vi "DataBase_Main.vi"(8 "error in (no error)":errorcluster) -> (0 "error out":errorcluster)   [LabVIEW 2020]
uses:
  Controller/#typedef_ControllerQueue_States.ctl
panel:
  out "appended path":path
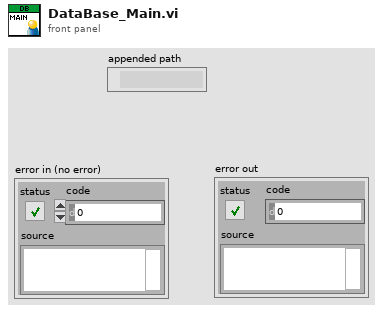
[diagram p1: front panel]
types:
  T1 = typedef "#typedef_ControllerQueue_States.ctl" = enum16{"Obtain", "GetRef", "Enqueue", "EnqueueAtOpp", "GetStatus", "Flush", "Release"}
  T2 = enum16{"open", "replace", "create", "open or create", "replace or create", "replace or create with confirmation"}
  T3 = typedef "#typedef_DataBase.ctl" = cluster{"Cmd":enum16{"Idle", "WriteLog", "Exit"}, "Temperature":dbl, "Logs":string}
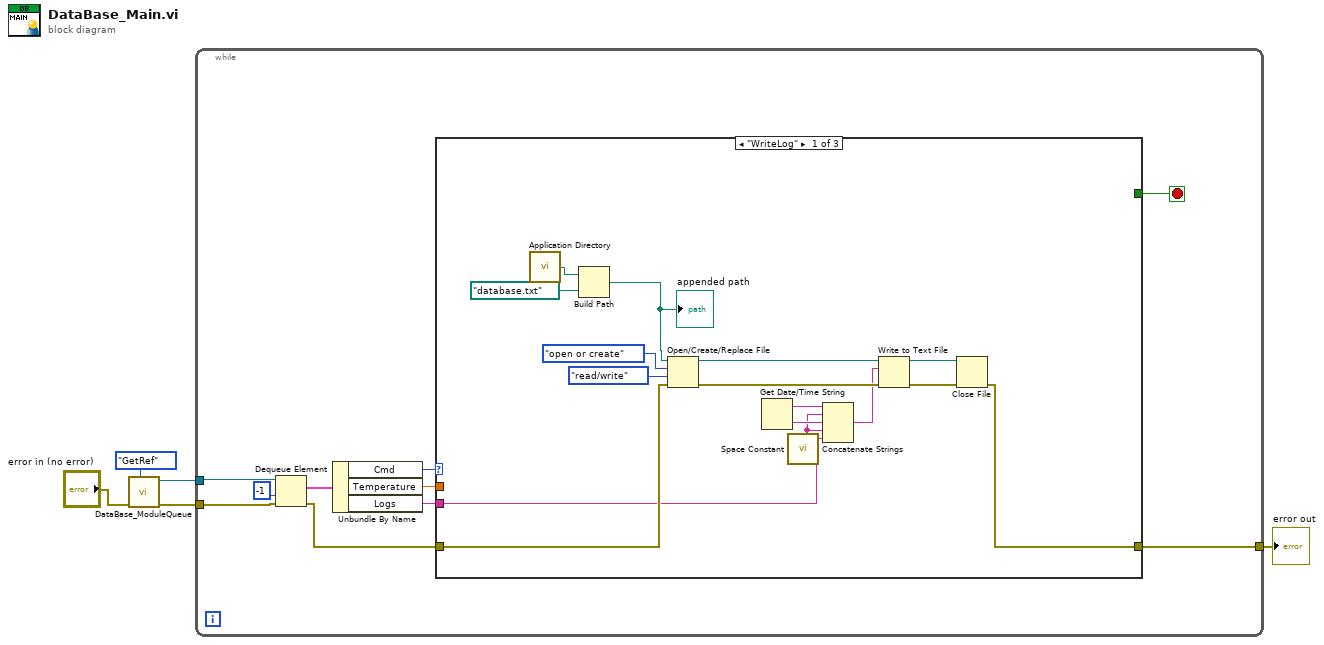
[diagram p0: block diagram]
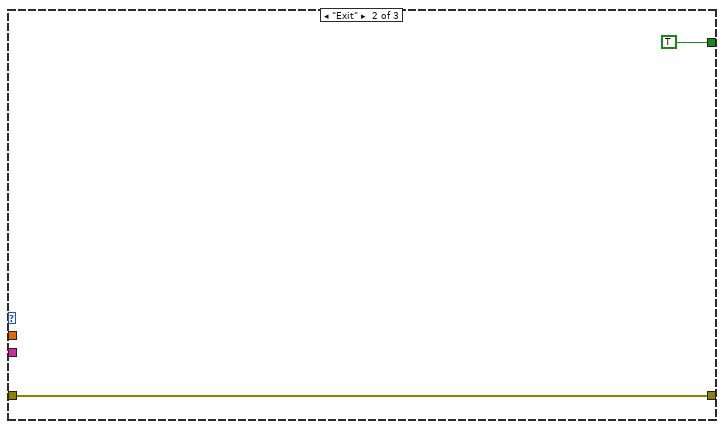
[diagram p2: hidden frame]
diagram:
  n1 = call "DataBase_ModuleQueue.vi"(7:#typedef_ControllerQueue_States."GetRef", "error in (no error)"="error in (no error)") -> ("error out"=w2:errorcluster, "queue out"=w3:refnum<queue>)  [unwired: 7 in, 1 out]
  n2 = while {
    tunnel: w3 -> [w13]
    tunnel: w2 -> [w14]
    tunnel: [w6] -> w1
    stop <- w8 stop-if-true
    n3 = Dequeue Element(queue=w13, timeout in ms (-1)=-1, error in (no error)=w14) -> (element=w12:T3, error out=w7:errorcluster)  [unwired: 2 out]
    n4 = Unbundle By Name(w12) -> ("Cmd"=w11:enum16{"Idle", "WriteLog", "Exit"}, "Temperature"=w10:dbl, "Logs"=w9:string)
    n5 = case shown="\"WriteLog\"" w11 {
      tunnel: w10 -> [_ _ _]
      tunnel: w9 -> [w16 _ _]
      tunnel: [_ TRUE _] -> w8
      tunnel: w7 -> [w29 w32 w34]
      tunnel: [w24 w32 w34] -> w6
      frame "WriteLog" {
        n6 = call <vilib>:"Application Directory.vi"() -> ("Application Directory"=w19:path)
        n7 = Build Path(base path=w19, name or relative path=path "database.txt") -> (appended path=w22:path)
        "appended path" <- w22
        n8 = Open/Create/Replace File(file path (use dialog)=w22, error in=w29, operation (0:open)=T2."open or create", access (0:read/write)=enum16{"read/write", "read-only", "write-only"}."read/write") -> (refnum out=w28:refnum<file>, error out=w25:errorcluster)  [unwired: 2 in, 1 out]
        n9 = Get Date/Time String() -> (date string=w21:string, time string=w18:string)  [unwired: 3 in]
        n10 = call <vilib>:"Space Constant.vi"() -> ("String"=w17:string)
        n11 = Concatenate Strings(w21, w17, w18, w17, w16) -> (w20:string)
        n12 = Write to Text File(file (use dialog)=w28, text=w20, error in=w25) -> (refnum out=w27:refnum<file>, error out=w26:errorcluster)  [unwired: 1 in, 1 out]
        n13 = Close File(refnum=w27, error in=w26) -> (error out=w24:errorcluster)  [unwired: 1 out]
      }
      frame "Exit" {
      }
      frame "Idle" {
      }
    }
  }
  "error out" <- w1
